vi "PeriodicTasksforSimulation.vi"(5 "Distance (Based on Encoder)":dbl, 7 "Gyro":dbl(knob) scale=-180.0..180.0, 8 "PID Constants":T4={"Drive Distance PID"={"proportional gain (Kc)"=1.0, "integral time (Ti, min)"=0.01, "derivative time (Td, min)"=0.0}, "Drive Straight PID"={"proportional gain (Kc)"=1.0, "integral time (Ti, min)"=0.01, "derivative time (Td, min)"=0.0}, "TurnPID"={"proportional gain (Kc)"=0.035, "integral time (Ti, min)"=0.0, "derivative time (Td, min)"=0.0008}, "Hold Position PID"={"proportional gain (Kc)"=0.2, "integral time (Ti, min)"=0.0, "derivative time (Td, min)"=0.001}} {"Hold Position PID"."derivative time (Td, min)" format="%.10f"; "Hold Position PID"."integral time (Ti, min)" format="%.8f"; "Hold Position PID"."proportional gain (Kc)" format="%.3f"; "TurnPID"."derivative time (Td, min)" format="%.6f"; "TurnPID"."integral time (Ti, min)" format="%.10f"; "TurnPID"."proportional gain (Kc)" format="%.6f"; "Drive Straight PID"."derivative time (Td, min)" format="%.6f"; "Drive Straight PID"."integral time (Ti, min)" format="%.10f"; "Drive Straight PID"."proportional gain (Kc)" format="%.6f"; "Drive Distance PID"."derivative time (Td, min)" format="%.10f"; "Drive Distance PID"."integral time (Ti, min)" format="%.8f"; "Drive Distance PID"."proportional gain (Kc)" format="%.3f"}, 9 "notifier out 2":refnum<notifier>, 10 "notifier out":refnum<notifier>, 11 "Tollerances":T2={"Evaluation Period"=0.5, "Dead Zone"=0.5, "Throttle Scale"=0.0}) -> (1 "Right Drive Motor":dbl, 2 "Left Drive Motor":dbl, 3 "Command":T3, 4 "Delta Angle Remaining":dbl, 6 "Distance Remaining":dbl)   [LabVIEW 2015]
uses:
  PID Constants.ctl
  Auto Control.ctl
  DriveStates.ctl
  Goal Selection.ctl
panel:
  out "Cheesy Steer":dbl
  out "Cheesy Throttle":dbl
  in  "Tab Control":enum32{"Turn Degree", "Page 2"}(tab)
  out "Angle":dbl
  out "Waveform Chart":T1(graph)
  out "Valid":bool
  out "Right Target":dbl
  out "Left Target":dbl
  out "Setpoint":dbl
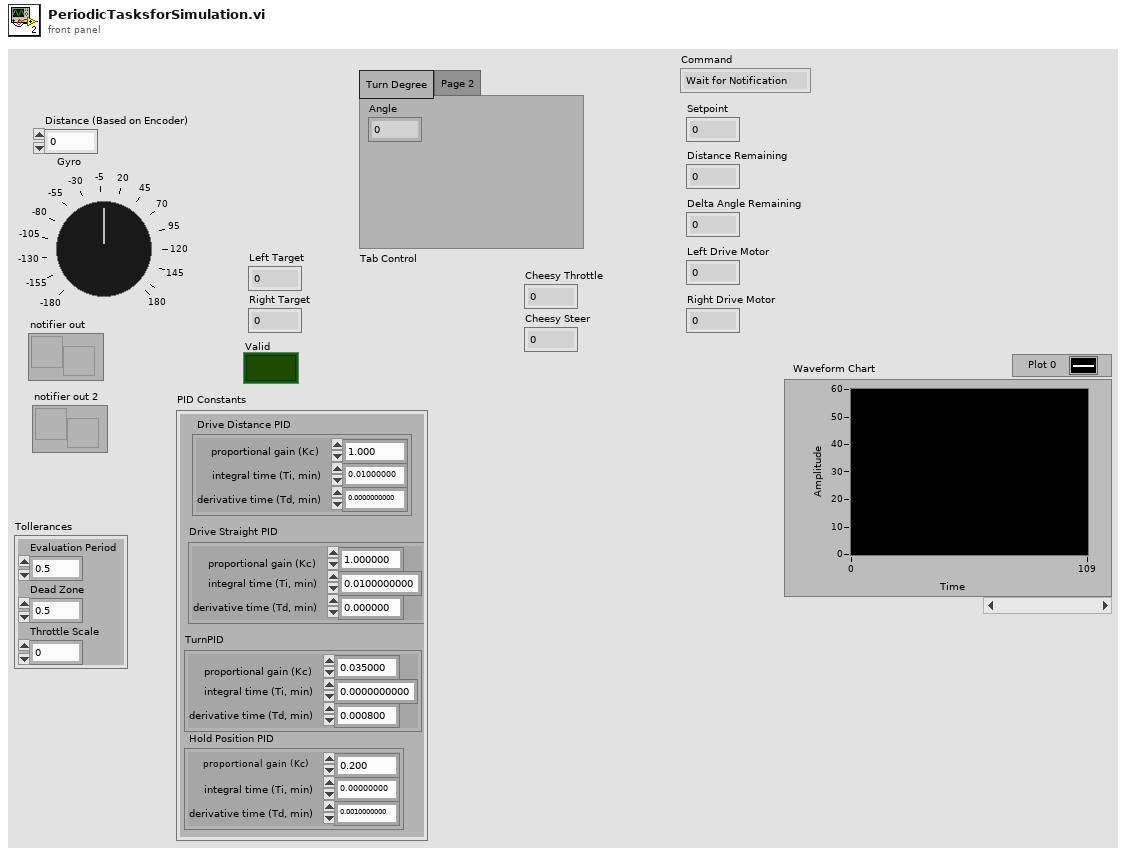
[diagram p1: front panel]
types:
  T1 = cluster{"Setpoint":dbl, "Delta Angle Remaining":dbl}
  T2 = cluster{"Evaluation Period":dbl, "Dead Zone":dbl, "Throttle Scale":dbl}
  T3 = typedef "DriveStates.ctl" = enum16{"Wait for Notification", "Drive for Distance", "Drive Continuous", "Drive Absolute Heading", "Drive Relative Heading", "Turn Continuous", "Turn Degree", "Stop", "Follow Camera", "Hold Position"}
  T4 = typedef "PID Constants.ctl" = cluster{"Drive Distance PID":cluster{"proportional gain (Kc)":dbl, "integral time (Ti, min)":dbl, "derivative time (Td, min)":dbl}, "Drive Straight PID":cluster{"proportional gain (Kc)":dbl, "integral time (Ti, min)":dbl, "derivative time (Td, min)":dbl}, "TurnPID":cluster{"proportional gain (Kc)":dbl, "integral time (Ti, min)":dbl, "derivative time (Td, min)":dbl}, "Hold Position PID":cluster{"proportional gain (Kc)":dbl, "integral time (Ti, min)":dbl, "derivative time (Td, min)":dbl}}
  T5 = cluster{"Delta":dbl, "Throttle Scale":dbl, "Current Angle":dbl, "Current Distance":dbl}
  T6 = typedef "Goal Selection.ctl" = enum16{"Left Goal", "Right Goal", "Stop"}
  T7 = typedef "Auto Control.ctl" = cluster{"Command":T3, "Distance":dbl, "Angle":dbl, "Power":dbl}
  T8 = cluster{"proportional gain (Kc)":dbl, "integral time (Ti, min)":dbl, "derivative time (Td, min)":dbl}
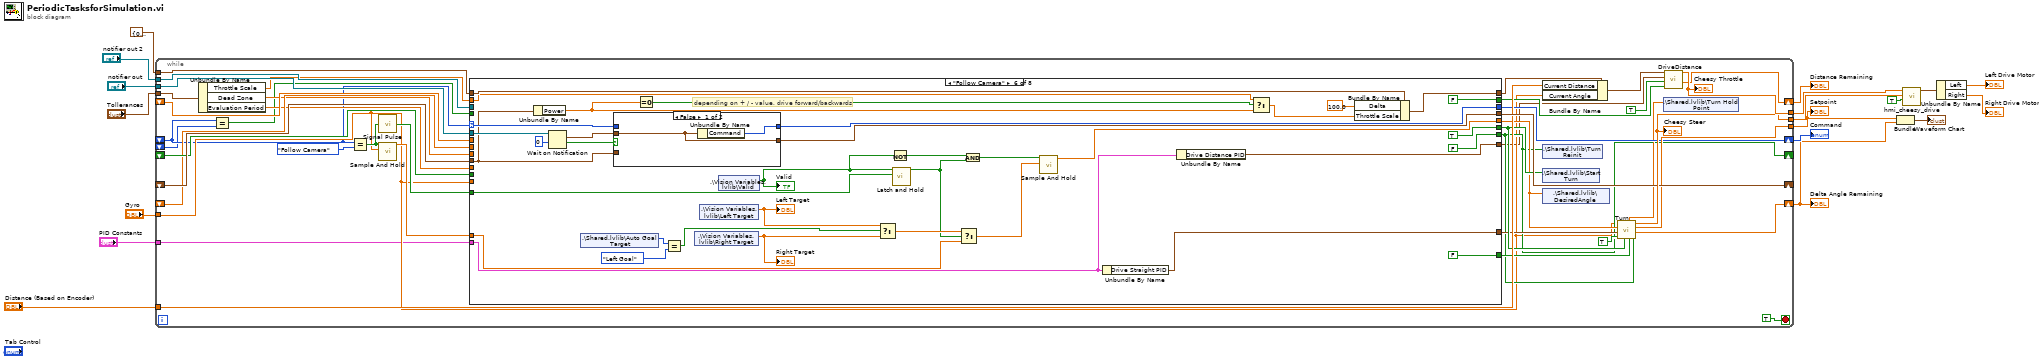
[diagram p0: block diagram]
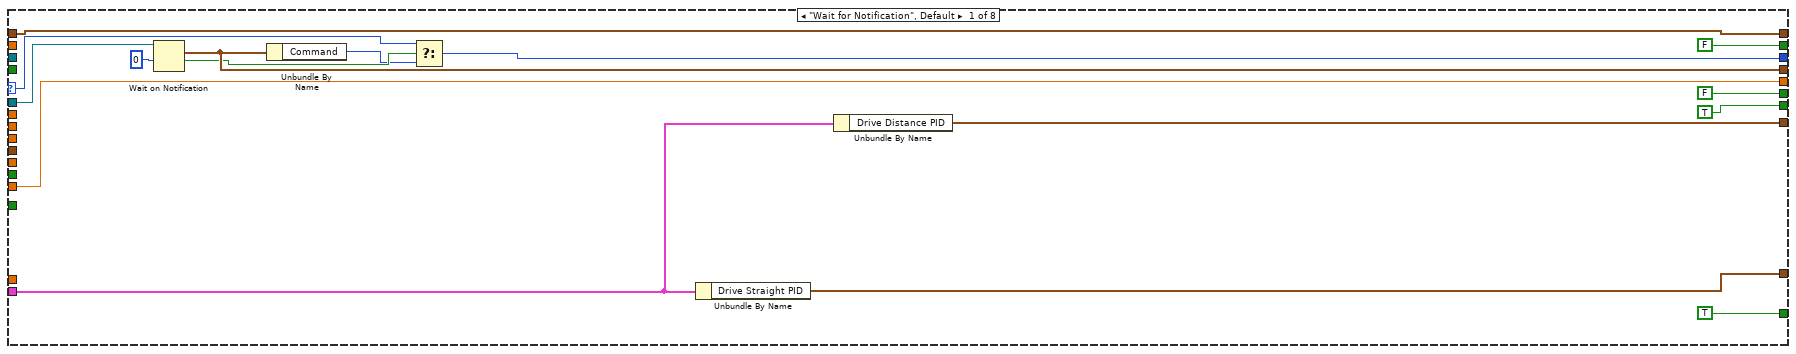
[diagram p2: hidden frame]
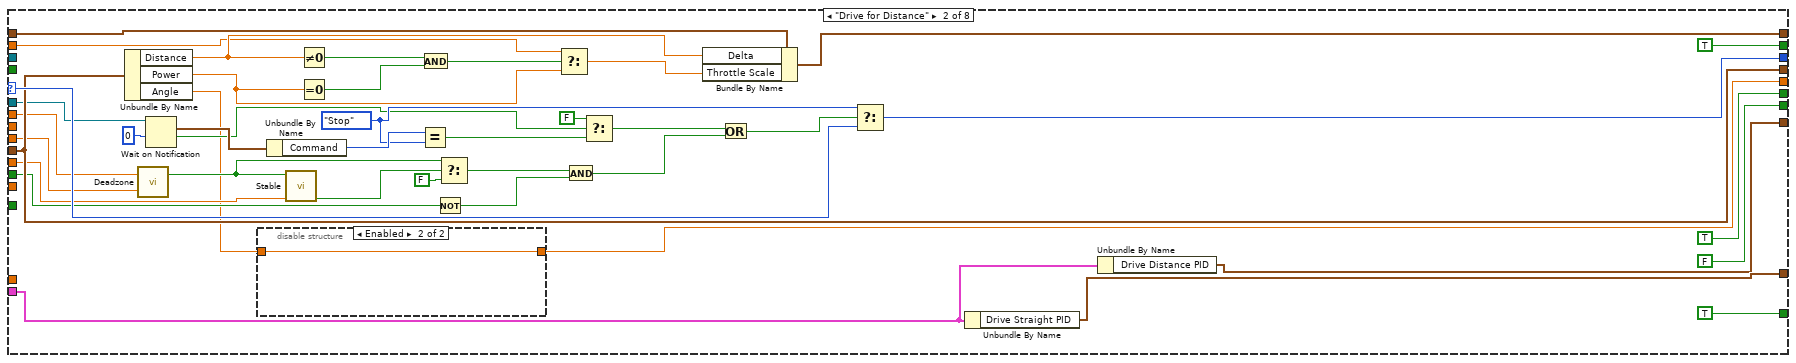
[diagram p3: hidden frame]
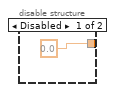
[diagram p4: hidden frame]
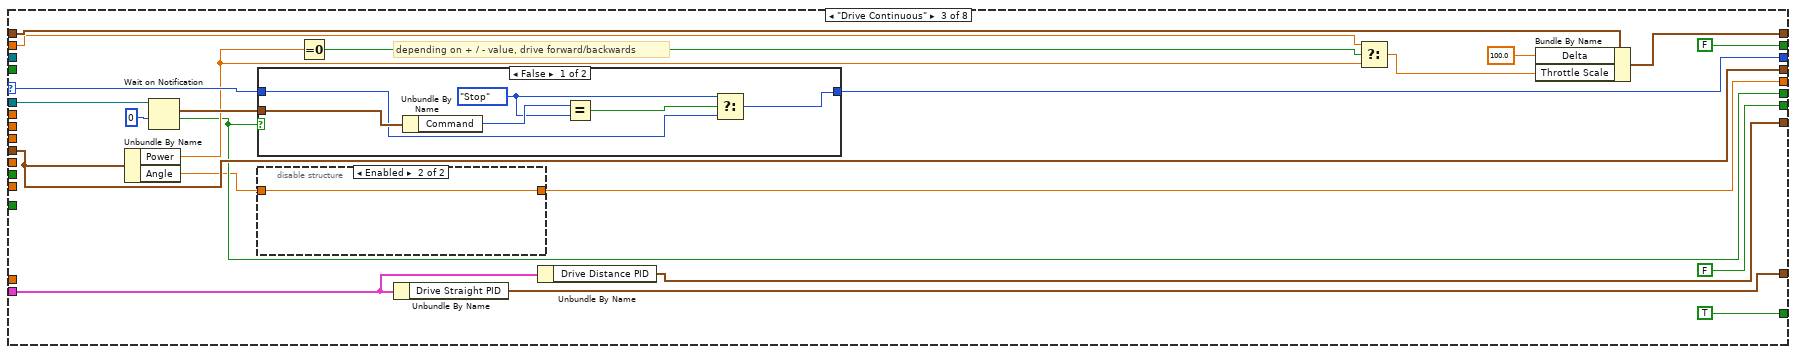
[diagram p5: hidden frame]
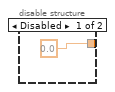
[diagram p6: hidden frame]
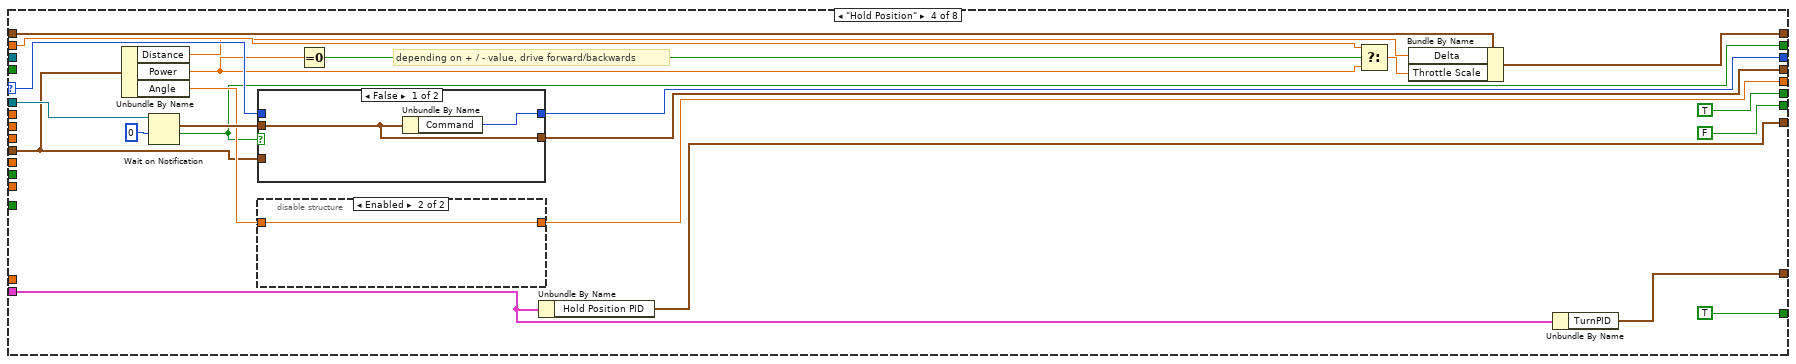
[diagram p8: hidden frame]
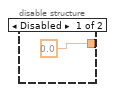
[diagram p9: hidden frame]
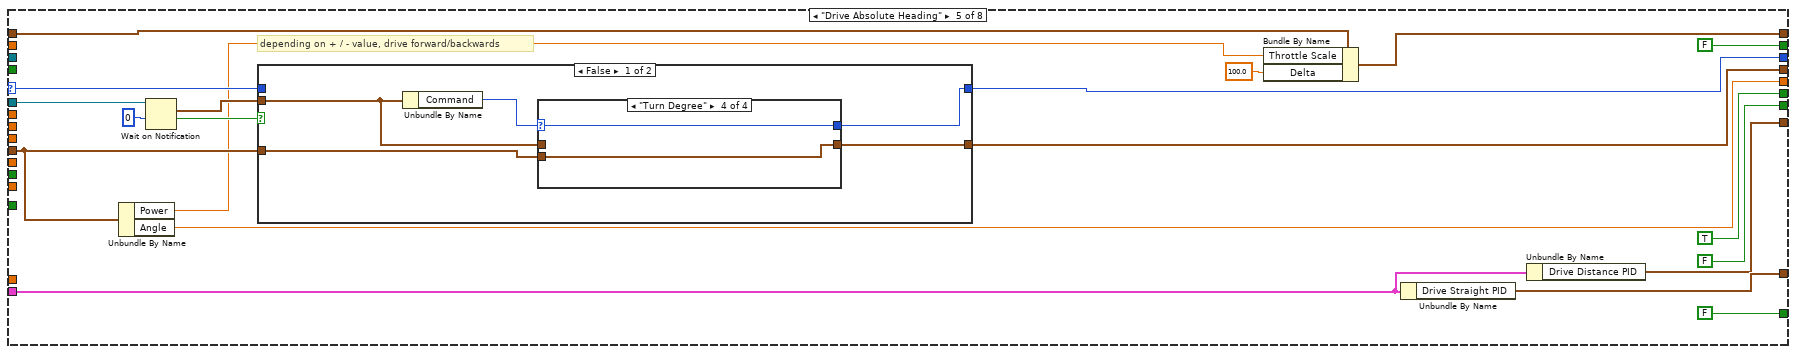
[diagram p11: hidden frame]
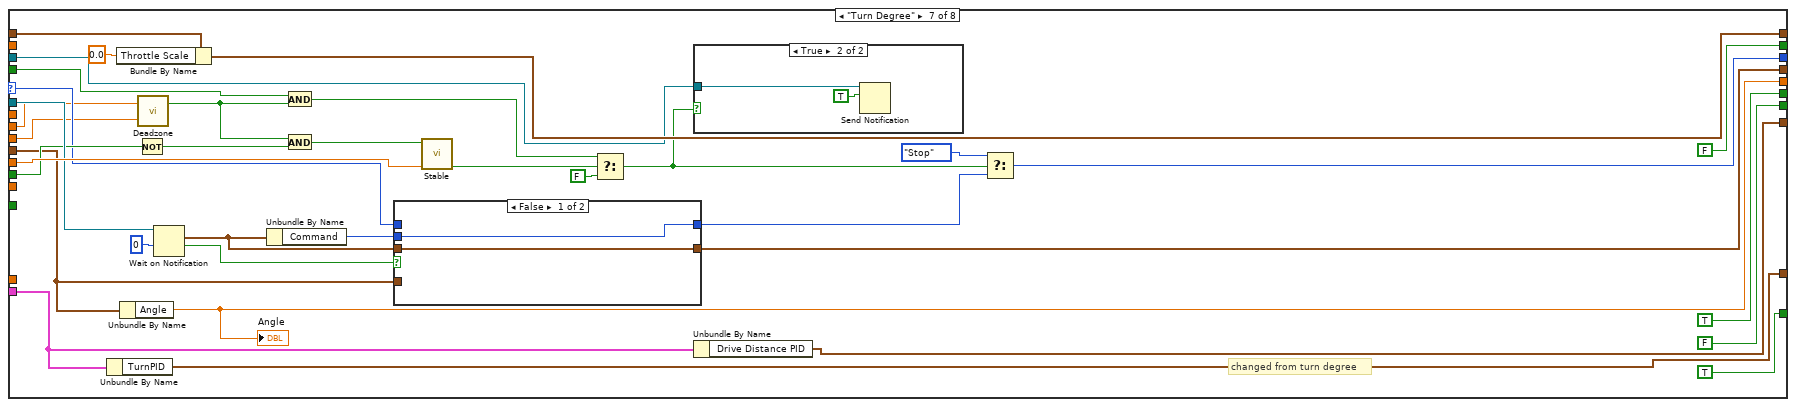
[diagram p17: hidden frame]
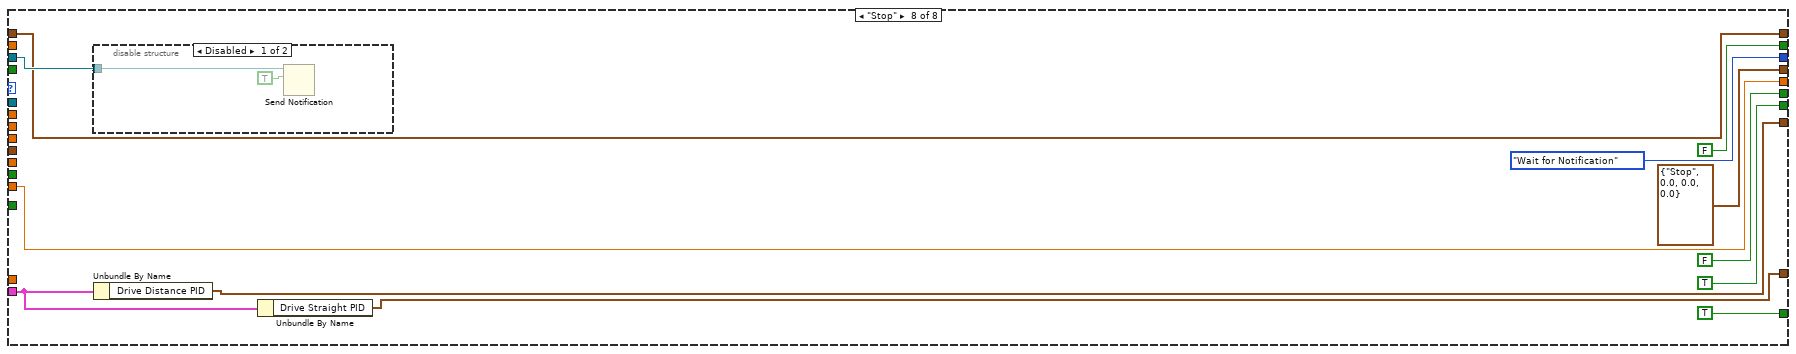
[diagram p20: hidden frame]
diagram:
  n1 = while {
    tunnel: "notifier out" -> [w56]
    tunnel: [w59] -> w18
    tunnel: [w58] -> w17
    tunnel: "notifier out 2" -> [w57]
    shift-right: [w27] -> w8
    shift-left: _ -> [w23]
    shift-right: [w53] -> _
    shift-left: _ -> [w54]
    tunnel: T5 {"Delta"=0.0, "Throttle Scale"=0.0, "Current Angle"=0.0, "Current Distance"=0.0} ("Drive Values 2") -> [w52]
    tunnel: "Gyro" -> [w24]
    tunnel: "Distance (Based on Encoder)" -> [w51]
    shift-right: [w25] -> _
    shift-left: _ -> [w50]
    shift-right: [w49] -> w4
    shift-left: _ -> [w48]
    shift-right: [w47] -> w1
    shift-left: _ -> [w46]
    tunnel: "Tollerances" -> [w41]
    tunnel: "PID Constants" -> [w20]
    tunnel: [w35] -> w2
    shift-left: _ -> [w22]
    stop <- TRUE stop-if-true
    n2 = Unbundle By Name(w41) -> ("Throttle Scale"=w39:dbl, "Dead Zone"=w40:dbl, "Evaluation Period"=w42:dbl)
    n3 = Equal?(x=w23, y=w22) -> (x = y?=w21:bool)
    n4 = Equal?(x=w23, y=DriveStates."Follow Camera" ("Command")) -> (x = y?=w31:bool)
    n5 = call <userlib>:"Signal Pulse.vi"("Input"=w31) -> ("Output"=w32:bool)
    n6 = call "Sample And Hold.vi"("Signal"=w24, "Condition"=w31) -> ("Signal Out"=w30:dbl)  [unwired: 9 in]
    n7 = case shown="\"Follow Camera\"" w23 {
      selector: w23 -> [w69 w111 w133 w165 w190 w241 w268 _]
      tunnel: [w68 w85 w132 w164 w189 w240 w283 DriveStates."Wait for Notification" ("Command")] -> w27
      tunnel: w57 -> [_ _ _ _ _ _ w257 w306]
      tunnel: w56 -> [w75 w91 w139 w171 w197 w248 w275 _]
      tunnel: [w71 w101 w128 w151 w185 w217 w264 T7 {"Command"=enum."Stop", "Distance"=0.0, "Angle"=0.0, "Power"=0.0} ("cluster")] -> w53
      tunnel: w52 -> [w66 w116 w140 w172 w198 w249 w286 w301]
      tunnel: [FALSE ("Start Turn") TRUE ("Start Turn") w122 TRUE ("Start Turn") TRUE ("Start Turn") TRUE ("Start Turn") TRUE ("Start Turn") FALSE ("Start Turn")] -> w43
      tunnel: [w62 w112 w135 w167 w184 w231 w279 w297] -> w28
      tunnel: [w66 w115 w137 w169 w195 w246 w285 w301] -> w44
      tunnel: [FALSE ("Start Drive Straight (Hold)") TRUE ("Start Drive Straight (Hold)") FALSE ("Start Drive Straight (Hold)") w155 FALSE ("Start Drive Straight (Hold)") FALSE ("Start Drive Straight (Hold)") FALSE ("Start Drive Straight (Hold)") FALSE ("Start Drive Straight (Hold)")] -> w34
      tunnel: w54 -> [_ w101 w128 w152 w186 w218 w266 _]
      tunnel: [TRUE FALSE FALSE FALSE FALSE FALSE FALSE TRUE] -> w25
      tunnel: w50 -> [_ w94 _ _ _ _ w272 _]
      tunnel: w48 -> [_ w100 _ _ _ _ _ _]
      tunnel: w46 -> [_ _ _ _ _ _ w262 _]
      tunnel: w42 -> [_ w97 _ _ _ _ w278 _]
      tunnel: w40 -> [_ w98 _ _ _ _ w254 _]
      tunnel: w39 -> [_ w96 w126 w159 _ w235 _ _]
      tunnel: [TRUE TRUE TRUE TRUE FALSE FALSE TRUE TRUE] -> w36
      tunnel: w32 -> [_ _ _ _ _ w228 _ _]
      tunnel: w30 -> [_ _ _ _ _ w222 _ _]
      tunnel: [w63 w79 w123 w157 w181 w221 w263 w298] -> w29
      tunnel: w20 -> [w61 w77 w120 w153 w180 w220 w255 w296]
      tunnel: w24 -> [w62 _ _ _ _ _ _ w297]
      tunnel: w21 -> [_ _ _ _ _ _ w259 _]
      tunnel: [w60 w76 w119 w154 w179 w219 w256 w295] -> w19
      frame "Wait for Notification", Default {
        n8 = Wait on Notification(notifier=w75, timeout in ms (-1)=0) -> (notification=w71:T7, timed out?=w70:bool)  [unwired: 2 in, 2 out]
        n9 = Unbundle By Name(w71) -> ("Command"=w67:T3)
        n10 = Select(t=w69, s=w70, f=w67) -> (s? t:f=w68:T3)
        n11 = Unbundle By Name(w61) -> ("Drive Straight PID"=w63:T8)
        n12 = Unbundle By Name(w61) -> ("Drive Distance PID"=w60:T8)
      }
      frame "Drive for Distance" {
        w88 = DriveStates."Stop" ("t")
        n13 = Unbundle By Name(w101) -> ("Distance"=w99:dbl, "Power"=w107:dbl, "Angle"=w78:dbl)
        n14 = call <userlib>:"Deadzone.vi"("Deadzone"=w98, "Input Signal"=w100) -> ("In Deadzone"=w104:bool)  [unwired: 1 out]
        n15 = Wait on Notification(notifier=w91, timeout in ms (-1)=0) -> (notification=w90:T7, timed out?=w84:bool)  [unwired: 2 in, 2 out]
        n16 = disable-structure shown="Enabled" {
          disable-tunnel: [0.0 ("Current Angle") w118] -> w112
          disable-tunnel: w78 -> [_ w118]
          frame Disabled {
          }
          frame Enabled {
          }
        }
        n17 = Unbundle By Name(w90) -> ("Command"=w89:T3)
        n18 = call <userlib>:"Stable.vi"("Eval Period (sec)"=w97, "Signal Input"=w104) -> ("Stable"=w105:bool)  [unwired: 9 in]
        n19 = Not Equal To 0?(x=w99) -> (x != 0?=w110:bool)
        n20 = Equal To 0?(x=w107) -> (x = 0?=w109:bool)
        n21 = Equal?(x=w89, y=w88) -> (x = y?=w83:bool)
        n22 = And(x=w110, y=w109) -> (x .and. y?=w108:bool)
        n23 = Not(x=w94) -> (.not. x?=w95:bool)
        n24 = Select(t=w104, s=w105, f=FALSE) -> (s? t:f=w93:bool)
        n25 = Select(t=w96, s=w108, f=w107) -> (s? t:f=w106:dbl)
        n26 = And(x=w93, y=w95) -> (x .and. y?=w87:bool)
        n27 = Select(t=FALSE, s=w84, f=w83) -> (s? t:f=w82:bool)
        n28 = Bundle By Name(cluster=w116, "Delta"=w99, "Throttle Scale"=w106) -> (w115:T5)
        n29 = Or(x=w82, y=w87) -> (x .or. y?=w86:bool)
        n30 = Select(t=w88, s=w86, f=w111) -> (s? t:f=w85:T3)
        n31 = Unbundle By Name(w77) -> ("Drive Straight PID"=w79:T8)
        n32 = Unbundle By Name(w77) -> ("Drive Distance PID"=w76:T8)
      }
      frame "Drive Continuous" {
        # "depending on + / - value, drive forward/backwards"
        n33 = Unbundle By Name(w128) -> ("Power"=w130:dbl, "Angle"=w121:dbl)
        n34 = Wait on Notification(notifier=w139, timeout in ms (-1)=0) -> (notification=w138:T7, timed out?=w122:bool)  [unwired: 2 in, 2 out]
        n35 = case shown="False" w122 {
          tunnel: w138 -> [w148 _]
          tunnel: [w146 w149] -> w132
          tunnel: w133 -> [w143 w149]
          frame False {
            w144 = DriveStates."Stop" ("y")
            n36 = Unbundle By Name(w148) -> ("Command"=w147:T3)
            n37 = Equal?(x=w147, y=w144) -> (x = y?=w145:bool)
            n38 = Select(t=w144, s=w145, f=w143) -> (s? t:f=w146:T3)
          }
          frame True {
          }
        }
        n39 = disable-structure shown="Enabled" {
          disable-tunnel: [0.0 ("Current Angle") w142] -> w135
          disable-tunnel: w121 -> [_ w142]
          frame Disabled {
          }
          frame Enabled {
          }
        }
        n40 = Equal To 0?(x=w130) -> (x = 0?=w131:bool)
        n41 = Unbundle By Name(w120) -> ("Drive Straight PID"=w123:T8)
        n42 = Unbundle By Name(w120) -> ("Drive Distance PID"=w119:T8)
        n43 = Select(t=w126, s=w131, f=w130) -> (s? t:f=w129:dbl)
        n44 = Bundle By Name(cluster=w140, "Delta"=100.0, "Throttle Scale"=w129) -> (w137:T5)
      }
      frame "Hold Position" {
        # "depending on + / - value, drive forward/backwards"
        n45 = Unbundle By Name(w152) -> ("Distance"=w150:dbl, "Power"=w162:dbl, "Angle"=w156:dbl)
        n46 = Wait on Notification(notifier=w171, timeout in ms (-1)=0) -> (notification=w170:T7, timed out?=w155:bool)  [unwired: 2 in, 2 out]
        n47 = case shown="False" w155 {
          tunnel: w170 -> [w175 _]
          tunnel: [w176 w178] -> w164
          tunnel: w165 -> [_ w178]
          tunnel: w152 -> [_ w177]
          tunnel: [w175 w177] -> w151
          frame False {
            n48 = Unbundle By Name(w175) -> ("Command"=w176:T3)
          }
          frame True {
          }
        }
        n49 = disable-structure shown="Enabled" {
          disable-tunnel: [0.0 ("Current Angle") w174] -> w167
          disable-tunnel: w156 -> [_ w174]
          frame Disabled {
          }
          frame Enabled {
          }
        }
        n50 = Equal To 0?(x=w162) -> (x = 0?=w163:bool)
        n51 = Unbundle By Name(w153) -> ("Hold Position PID"=w154:T8)
        n52 = Select(t=w159, s=w163, f=w162) -> (s? t:f=w161:dbl)
        n53 = Bundle By Name(cluster=w172, "Delta"=w150, "Throttle Scale"=w161) -> (w169:T5)
        n54 = Unbundle By Name(w153) -> ("TurnPID"=w157:T8)
      }
      frame "Drive Absolute Heading" {
        # "depending on + / - value, drive forward/backwards"
        n55 = Unbundle By Name(w186) -> ("Power"=w182:dbl, "Angle"=w184:dbl)
        n56 = Wait on Notification(notifier=w197, timeout in ms (-1)=0) -> (notification=w196:T7, timed out?=w191:bool)  [unwired: 2 in, 2 out]
        n57 = case shown="False" w191 {
          tunnel: w196 -> [w199 _]
          tunnel: [w203 w213] -> w189
          tunnel: w190 -> [_ w213]
          tunnel: w186 -> [w201 w212]
          tunnel: [w200 w212] -> w185
          frame False {
            n58 = Unbundle By Name(w199) -> ("Command"=w202:T3)
            n59 = case shown="\"Turn Degree\"" w202 {
              selector: w202 -> [w204 w207 w209 w211]
              tunnel: [w204 w207 w209 w211] -> w203
              tunnel: w201 -> [_ w206 _ w210]
              tunnel: [w205 w206 w208 w210] -> w200
              tunnel: w199 -> [w205 _ w208 _]
              frame "Drive Absolute Heading" {
              }
              frame "Stop", Default {
              }
              frame "Follow Camera" {
              }
              frame "Turn Degree" {
              }
            }
          }
          frame True {
          }
        }
        n60 = Bundle By Name(cluster=w198, "Throttle Scale"=w182, "Delta"=100.0) -> (w195:T5)
        n61 = Unbundle By Name(w180) -> ("Drive Straight PID"=w181:T8)
        n62 = Unbundle By Name(w180) -> ("Drive Distance PID"=w179:T8)
      }
      frame "Follow Camera" {
        # "depending on + / - value, drive forward/backwards"
        n63 = Unbundle By Name(w218) -> ("Power"=w238:dbl)
        n64 = Wait on Notification(notifier=w248, timeout in ms (-1)=0) -> (notification=w247:T7, timed out?=w242:bool)  [unwired: 2 in, 2 out]
        n65 = shared-variable ".\\Shared.lvlib\\Auto Goal Target"() -> (w216:enum16{"Left Goal", "Right Goal", "Stop"})  [unwired: 1 in, 1 out]
        n66 = case shown="False" w242 {
          tunnel: w247 -> [w250 _]
          tunnel: [w251 w253] -> w240
          tunnel: w241 -> [_ w253]
          tunnel: w218 -> [_ w252]
          tunnel: [w250 w252] -> w217
          frame False {
            n67 = Unbundle By Name(w250) -> ("Command"=w251:T3)
          }
          frame True {
          }
        }
        n68 = Equal To 0?(x=w238) -> (x = 0?=w239:bool)
        n69 = Equal?(x=w216, y=Goal_Selection."Left Goal" ("Goal Target")) -> (x = y?=w214:bool)
        n70 = shared-variable ".\\Vision Variables.lvlib\\Right Target"() -> (w234:dbl)  [unwired: 1 in, 1 out]
        "Right Target" <- w234
        n71 = shared-variable ".\\Vision Variables.lvlib\\Left Target"() -> (w233:dbl)  [unwired: 1 in, 1 out]
        "Left Target" <- w233
        n72 = shared-variable ".\\Vision Variables.lvlib\\Valid"() -> (w229:bool)  [unwired: 1 in, 1 out]
        "Valid" <- w229
        n73 = Select(t=w233, s=w214, f=w234) -> (s? t:f=w225:dbl)
        n74 = Not(x=w229) -> (.not. x?=w227:bool)
        n75 = call "Latch and Hold.vi"("Clear"=w228, "Valid"=w229) -> ("Output"=w224:bool)  [unwired: 9 in]
        n76 = Select(t=w225, s=w224, f=w222) -> (s? t:f=w223:dbl)
        n77 = And(x=w227, y=w224) -> (x .and. y?=w226:bool)
        n78 = call "Sample And Hold.vi"("Signal"=w223, "Condition"=w226) -> ("Signal Out"=w231:dbl)  [unwired: 9 in]
        n79 = Unbundle By Name(w220) -> ("Drive Straight PID"=w221:T8)
        n80 = Unbundle By Name(w220) -> ("Drive Distance PID"=w219:T8)
        n81 = Select(t=w235, s=w239, f=w238) -> (s? t:f=w237:dbl)
        n82 = Bundle By Name(cluster=w249, "Delta"=100.0, "Throttle Scale"=w237) -> (w246:T5)
      }
      frame "Turn Degree" {
        # "changed from turn degree"
        n83 = Unbundle By Name(w255) -> ("TurnPID"=w263:T8)
        n84 = Bundle By Name(cluster=w286, "Throttle Scale"=0.0) -> (w285:T5)
        n85 = Unbundle By Name(w266) -> ("Angle"=w279:dbl)
        "Angle" <- w279
        n86 = Not(x=w272) -> (.not. x?=w271:bool)
        n87 = call <userlib>:"Deadzone.vi"("Deadzone"=w254, "Input Signal"=w262) -> ("In Deadzone"=w261:bool)  [unwired: 1 out]
        n88 = Wait on Notification(notifier=w275, timeout in ms (-1)=0) -> (notification=w265:T7, timed out?=w270:bool)  [unwired: 2 in, 2 out]
        n89 = Unbundle By Name(w265) -> ("Command"=w269:T3)
        n90 = And(x=w259, y=w261) -> (x .and. y?=w260:bool)
        n91 = And(x=w261, y=w271) -> (x .and. y?=w273:bool)
        n92 = case shown="False" w270 {
          tunnel: w269 -> [w292 _]
          tunnel: w268 -> [_ w294]
          tunnel: [w292 w294] -> w267
          tunnel: w266 -> [_ w293]
          tunnel: w265 -> [w291 _]
          tunnel: [w291 w293] -> w264
          frame False {
          }
          frame True {
          }
        }
        n93 = call <userlib>:"Stable.vi"("Eval Period (sec)"=w278, "Signal Input"=w273) -> ("Stable"=w281:bool)  [unwired: 9 in]
        n94 = Select(t=w260, s=w281, f=FALSE) -> (s? t:f=w258:bool)
        n95 = case shown="True" w258 {
          tunnel: w257 -> [_ w289]
          frame False {
          }
          frame True {
            n96 = Send Notification(notification=TRUE, notifier=w289) -> ()  [unwired: 1 in, 2 out]
          }
        }
        n97 = Unbundle By Name(w255) -> ("Drive Distance PID"=w256:T8)
        n98 = Select(t=DriveStates."Stop", s=w258, f=w267) -> (s? t:f=w283:T3)
      }
      frame "Stop" {
        n99 = disable-structure shown="Disabled" {
          disable-tunnel: w306 -> [w308 _]
          frame Disabled {
            n100 = Send Notification(notification=TRUE, notifier=w308) -> ()  [unwired: 1 in, 2 out]
          }
          frame Enabled {
          }
        }
        n101 = Unbundle By Name(w296) -> ("Drive Distance PID"=w295:T8)
        n102 = Unbundle By Name(w296) -> ("Drive Straight PID"=w298:T8)
      }
    }
    n103 = Bundle By Name(cluster=w44, "Current Distance"=w51, "Current Angle"=w24) -> (w45:T5)
    n104 = shared-variable ".\\Shared.lvlib\\Turn Reinit"(w25) -> ()  [unwired: 1 in, 1 out]
    n105 = shared-variable ".\\Shared.lvlib\\Start Turn"(w43) -> ()  [unwired: 1 in, 1 out]
    n106 = shared-variable ".\\Shared.lvlib\\DesiredAngle"(w28) -> ()  [unwired: 1 in, 1 out]
    n107 = call "Turn.vi"("reinitialize?"=w25, "Delta?"=w36, "Start Turn"=w43, "Negate"=TRUE, "PID gains"=w29, "Desired Angle"=w28, "Current Angle"=w24) -> ("Delta Angle Remaining"=w47:dbl, "Setpoint"=w35:dbl, "Cheesy Steer"=w58:dbl, "Turn Hold Point"=w26:dbl)  [unwired: 1 in]
    "Cheesy Steer" <- w58
    n108 = shared-variable ".\\Shared.lvlib\\Turn Hold Point"(w26) -> ()  [unwired: 1 in, 1 out]
    n109 = call "DriveDistance.vi"("Start Drive Straight (Hold)"=w34, "Negate"=TRUE, "Drive PID"=w19, "Drive Values"=w45) -> ("Distance Remaining"=w49:dbl, "Cheesy Throttle"=w59:dbl)  [unwired: 6 in]
    "Cheesy Throttle" <- w59
  }
  "Command" <- w8
  "Delta Angle Remaining" <- w1
  "Distance Remaining" <- w4
  "Setpoint" <- w2
  n110 = Bundle("Setpoint"=w2, "Delta Angle Remaining"=w1) -> (→"Waveform Chart":T1)  [unwired: 1 in]
  n111 = call <userlib>:"hmi_cheesy_drive.vi"("Quick Turn"=TRUE, "Wheel"=w17, "Throttle"=w18) -> ("Drive Data"=w16:cluster{"Left":dbl, "Right":dbl})  [unwired: 8 in]
  n112 = Unbundle By Name(w16) -> ("Left"=→"Left Drive Motor":dbl, "Right"=→"Right Drive Motor":dbl)
